vi "zad_7.vi"() -> ()   [LabVIEW 2025]
panel:
  out "error out":errorcluster
  out "XY Graph":cluster{i32[], dbl[]}[](graph)
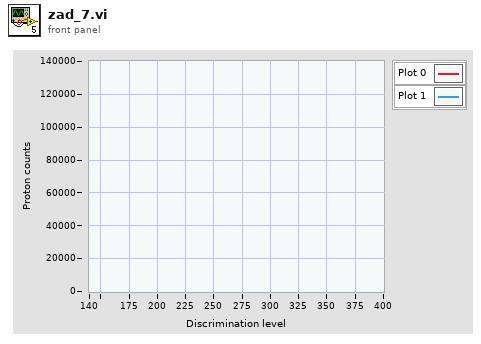
[diagram p1: front panel]
types:
  T1 = enum16{"big-endian, network order", "native, host order", "little-endian"}
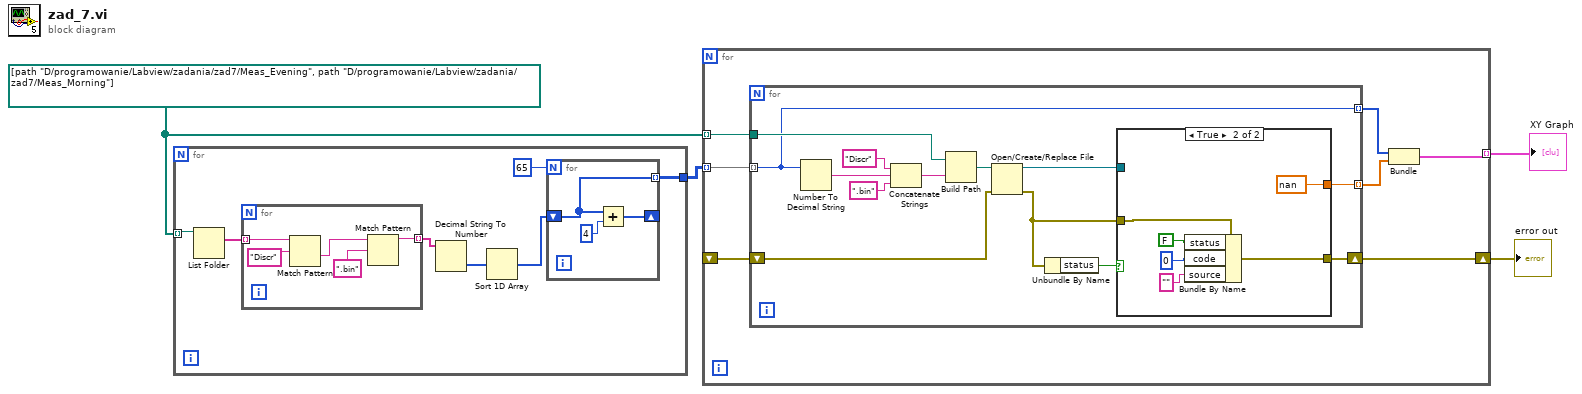
[diagram p0: block diagram]
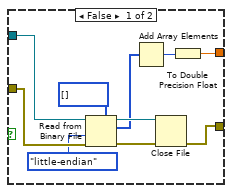
[diagram p2: hidden frame]
diagram:
  w2 = path[] [path "D:/programowanie/Labview/zadania/zad7/Meas_Evening", path "D:/programowanie/Labview/zadania/zad7/Meas_Morning"]
  n1 = for {
    tunnel: w2 -> [w11] mode=indexing
    tunnel: [w6] -> w1
    n2 = List Folder(path=w11) -> (filenames=w10:string[])  [unwired: 3 in, 3 out]
    n3 = for {
      tunnel: w10 -> [w19] mode=indexing
      tunnel: [w15] -> w9 mode=indexing
      n4 = Match Pattern(string=w19, regular expression="Discr") -> (after substring=w17:string)  [unwired: 1 in, 3 out]
      n5 = Match Pattern(string=w17, regular expression=".bin") -> (before substring=w15:string)  [unwired: 1 in, 3 out]
    }
    n6 = Decimal String To Number(string=w9) -> (number=w8:i32[])  [unwired: 2 in, 1 out]
    n7 = Sort 1D Array(array=w8) -> (sorted array=w5:i32[])
    n8 = for {
      N: 65 -> [_]
      shift-right: [w14] -> _
      shift-left: w5 -> [w12]
      tunnel: [w12] -> w6 mode=indexing
      n9 = Add(x=w12, y=4 ("x")) -> (x+y=w14:i32[])
    }
  }
  n10 = for {
    tunnel: w2 -> [w26] mode=indexing
    tunnel: w1 -> [w25] mode=indexing
    shift-right: [w23] -> w4
    shift-left: _ -> [w22]
    tunnel: [w20] -> w3 mode=indexing
    n11 = for {
      tunnel: w26 -> [w38]
      tunnel: w25 -> [w31] mode=indexing
      tunnel: [w32] -> w21 mode=indexing
      tunnel: [w31] -> w24 mode=indexing
      shift-right: [w30] -> w23
      shift-left: w22 -> [w29]
      n12 = Number To Decimal String(number=w31) -> (decimal integer string=w37:string)  [unwired: 1 in]
      n13 = Concatenate Strings("Discr" ("string"), w37, ".bin" ("string")) -> (w34:string)
      n14 = Build Path(base path=w38, name or relative path=w34) -> (appended path=w39:path)
      n15 = Open/Create/Replace File(file path (use dialog)=w39, error in=w29) -> (refnum out=w33:refnum<file>, error out=w28:errorcluster)  [unwired: 4 in, 1 out]
      n16 = Unbundle By Name(w28) -> ("status"=w27:bool)
      n17 = case shown="True" w27 {
        tunnel: w33 -> [w49 _]
        tunnel: [w43 nan] -> w32
        tunnel: [w45 w50] -> w30
        tunnel: w28 -> [w48 w54]
        frame False {
          n18 = Read from Binary File(5:u32[] [], 8:w48, 9:T1."little-endian" ("byte order (0:big-endian, network order)"), 11:w49) -> (0:w47:errorcluster, 2:w41:u32[], 3:w46:refnum<file>)  [unwired: 2 in, 1 out]
          n19 = Add Array Elements(numeric array=w41) -> (sum=w40:u32)
          n20 = Close File(refnum=w46, error in=w47) -> (error out=w45:errorcluster)  [unwired: 1 out]
          n21 = To Double Precision Float(number=w40) -> (double precision float=w43:dbl)
        }
        frame True {
          n22 = Bundle By Name(cluster=w54, "status"=FALSE, "code"=0, "source"="") -> (w50:errorcluster)
        }
      }
    }
    n23 = Bundle(w24, w21) -> (w20:cluster{i32[], dbl[]})  [unwired: 1 in]
  }
  "XY Graph" <- w3
  "error out" <- w4
